vi "DeriveParameters.vi"(8 "error in (no error)":errorcluster, 9 "Parameters":T2={"number of planes"=4, "z step"=1.9999999999999998e-05, "pixel dwell time"=1.0000000000000001e-11, "z frequency"=10.0, "number of pixels"=100, "smooth points"=10, "smooth line"=10, "Sine\nSawtooth"=FALSE, "PointSorting"=0, "Sort Points"=FALSE, "X-pixels"=256.0, "Y-lines"=256.0, "pixelstoµm"=256.0, "zoom"=1.0, "Time offset"=1.0000000000000001e-11} {"zoom" min=0.5 step=0.1; "Y-lines" min=1 step=1; "X-pixels" min=1 step=1; "PointSorting" items=["No Difference", "Every Second Point", "Down / Up"]; "smooth line" min=1; "smooth points" min=1; "number of pixels" min=1; "z frequency" format="%_4g"; "number of planes" min=1}, 10 "DutyCluster":T1 {"Iteration" items=["first iteration", "second iteration"]}, 11 "XYZ Point coordinates (pixels)":dbl[][](array[numeric])) -> (0 "error out":errorcluster, 2 "DutyCluster":T1 {"Iteration" items=["first iteration", "second iteration"]})   [LabVIEW 2010]
uses:
  TypeDefs/DutyCluster.ctl
  TypeDefs/ParameterCluster.ctl
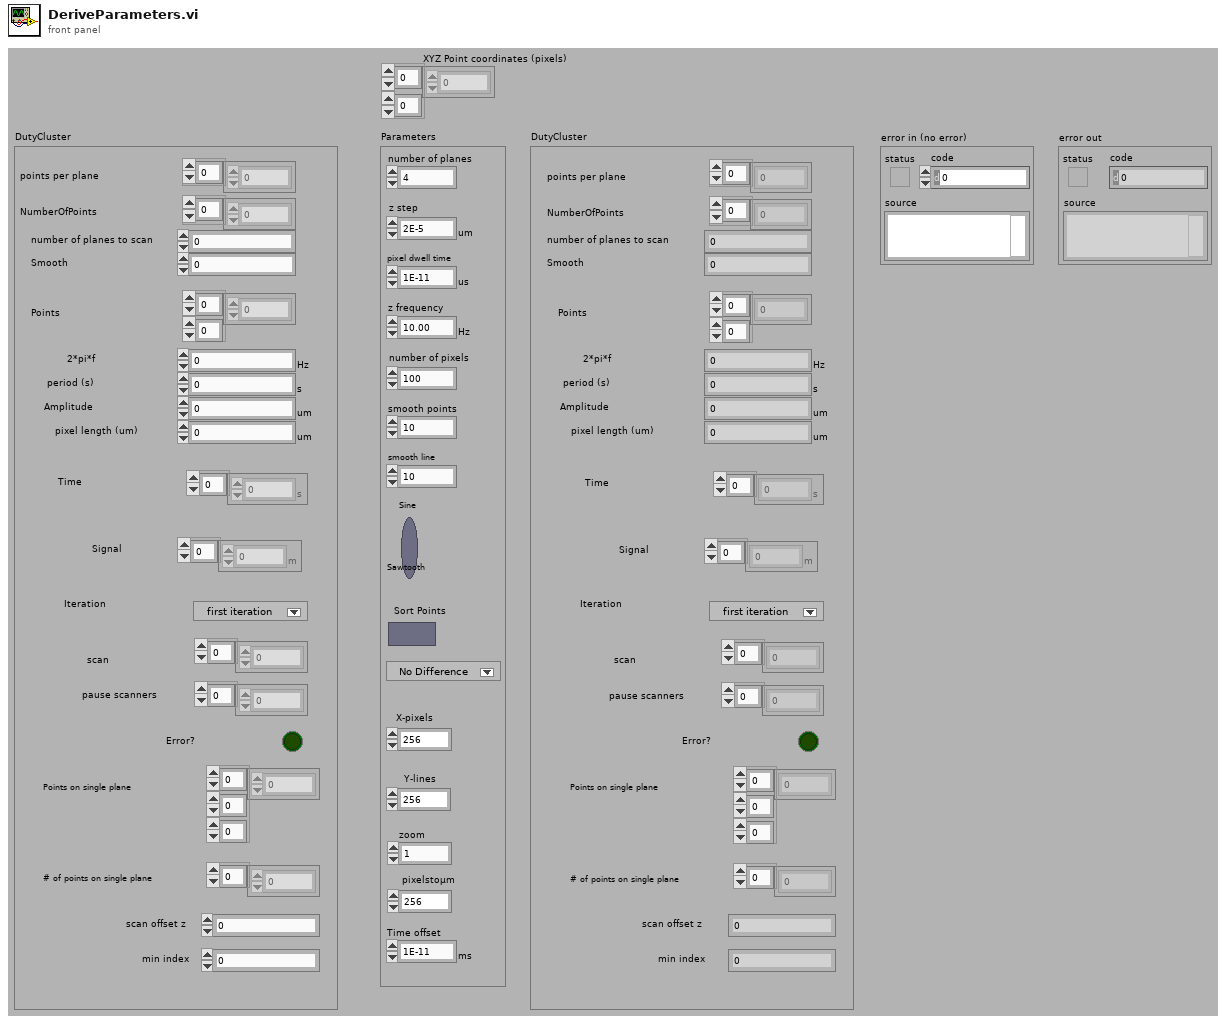
[diagram p1: front panel]
types:
  T1 = typedef "DutyCluster.ctl" = cluster{"points per plane":i32[], "NumberOfPoints":i32[], "number of planes to scan":i32, "Smooth":i32, "Points":dbl[][], "2*pi*f":dbl[unit], "period (s)":dbl[unit], "Amplitude":dbl[unit], "pixel length (um)":dbl[unit], "Time":dbl[unit][], "Signal":dbl[unit][], "Iteration":u16, "scan":i32[], "pause scanners":i32[], "Error?":bool, "Points on single plane":dbl[][][], "# of points on single plane":i32[], "scan offset z":i32, "min index":i32}
  T2 = typedef "ParameterCluster.ctl" = cluster{"number of planes":i32, "z step":dbl[unit], "pixel dwell time":dbl[unit], "z frequency":dbl[unit], "number of pixels":i32, "smooth points":i32, "smooth line":i32, "Sine\nSawtooth":bool, "PointSorting":u16, "Sort Points":bool, "X-pixels":sgl, "Y-lines":sgl, "pixelstoµm":dbl, "zoom":dbl, "Time offset":dbl[unit]}
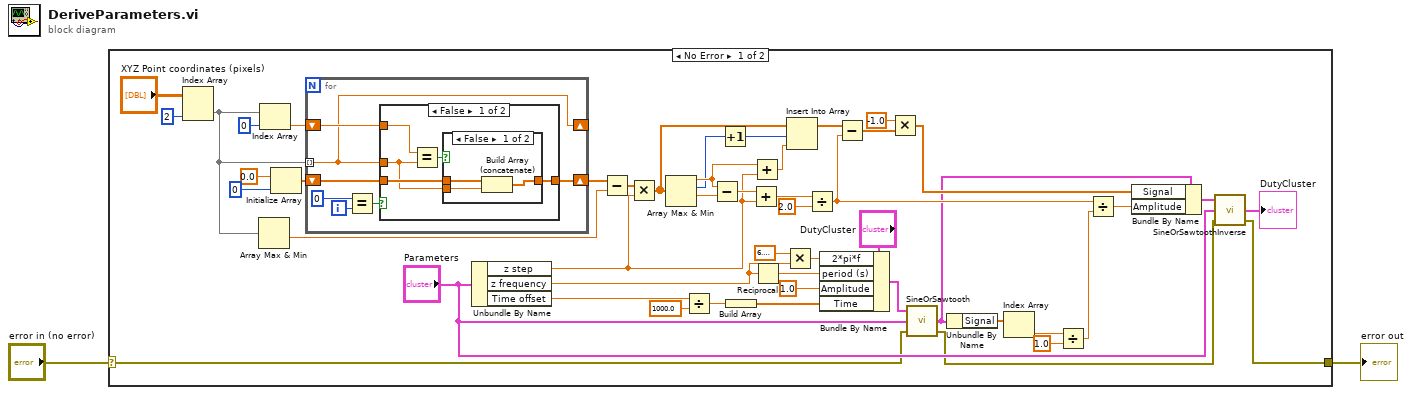
[diagram p0: block diagram]
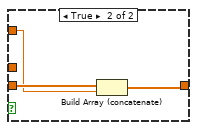
[diagram p3: hidden frame]
diagram:
  n1 = case shown="No Error" "error in (no error)" {
    selector: "error in (no error)" -> [w8 w71]
    tunnel: [w7 w71] -> w1
    frame No Error {
      n2 = Index Array(array="XYZ Point coordinates (pixels)", index (col)=2 ("disabled index (col)")) -> (element=w4:dbl[])  [unwired: 1 in]
      n3 = Array Max & Min(array=w4) -> (min value=w28:dbl)  [unwired: 3 out]
      n4 = Index Array(array=w4, index=0) -> (element=w47:dbl)
      n5 = Initialize Array(0.0 ("element"), 0 ("dimension size")) -> (w49:dbl[])
      n6 = for {
        tunnel: w4 -> [w52] mode=indexing
        shift-right: [w52] -> _
        shift-left: w47 -> [w56]
        shift-right: [w57] -> w3
        shift-left: w49 -> [w58]
        i -> [w55]
        n7 = Equal?(x=0, y=w55) -> (x = y?=w53:bool)
        n8 = case shown="False" w53 {
          tunnel: w58 -> [w62 w70]
          tunnel: [w61 w68] -> w57
          tunnel: w56 -> [w60 w69]
          tunnel: w52 -> [w59 _]
          frame False {
            n9 = Equal?(x=w60, y=w59) -> (x = y?=w63:bool)
            n10 = case shown="False" w63 {
              tunnel: w62 -> [w65 w67]
              tunnel: [w64 w67] -> w61
              tunnel: w59 -> [w66 _]
              frame False {
                n11 = Build Array (concatenate)(w65, w66) -> (w64:dbl[])
              }
              frame True {
              }
            }
          }
          frame True {
            n12 = Build Array (concatenate)(w70, w69) -> (w68:dbl[])
          }
        }
      }
      n13 = Unbundle By Name("Parameters") -> ("z step"=w27:dbl[unit], "z frequency"=w26:dbl[unit], "Time offset"=w25:dbl[unit])
      n14 = Subtract(x=w3, y=w28) -> (x-y=w31:dbl[])
      n15 = Multiply(x=w31, y=w27) -> (x*y=w39:dbl[unit][])
      n16 = Array Max & Min(array=w39) -> (max value=w38:dbl[unit], max index (indices)=w36:i32, min value=w46:dbl[unit])  [unwired: 1 out]
      n17 = Divide(x=w25, y=1000.0) -> (x/y=w30:dbl[unit])
      n18 = Subtract(x=w38, y=w46) -> (x-y=w41:dbl[unit])
      n19 = Increment(x=w36) -> (x+1=w37:i32)
      n20 = Build Array(w30) -> (w10:dbl[unit][])
      n21 = Add(x=w41, y=w27) -> (x+y=w42:dbl[unit])
      n22 = Add(x=w38, y=w27) -> (x+y=w35:dbl[unit])
      n23 = Reciprocal(x=w26) -> (1/x=w24:dbl[unit])
      n24 = Multiply(x=6.283185307179586, y=w26) -> (x*y=w23:dbl[unit])
      n25 = Insert Into Array(array=w39, index=w37, new element=w35) -> (w34:dbl[unit][])
      n26 = Divide(x=w42, y=2.0) -> (x/y=w40:dbl[unit])
      n27 = Bundle By Name(cluster="DutyCluster", "2*pi*f"=w23, "period (s)"=w24, "Amplitude"=dbl[unit] 1.0, "Time"=w10) -> (w12:T1)
      n28 = Subtract(x=w34, y=w40) -> (x-y=w32:dbl[unit][])
      n29 = Multiply(x=-1.0 ("y"), y=w32) -> (x*y=w16:dbl[unit][])
      n30 = call "SineOrSawtooth.vi"("error in (no error)"=w8, "Parameters"="Parameters", "DutyCluster"=w12) -> ("error out"=w9:errorcluster, "DutyCluster"=w5:T1)  [unwired: 1 in]
      n31 = Unbundle By Name(w5) -> ("Signal"=w17:dbl[unit][])
      n32 = Index Array(array=w17) -> (element=w19:dbl[unit])  [unwired: 1 in]
      n33 = Divide(x=w19, y=dbl[unit] 1.0) -> (x/y=w18:dbl)
      n34 = Divide(x=w40, y=w18) -> (x/y=w22:dbl[unit])
      n35 = Bundle By Name(cluster=w5, "Signal"=w16, "Amplitude"=w22) -> (w15:T1)
      n36 = call "SineOrSawtoothInverse.vi"("error in (no error)"=w9, "Parameters"="Parameters", "DutyCluster"=w15) -> ("error out"=w7:errorcluster, "DutyCluster"=→"DutyCluster":T1)  [unwired: 1 in]
    }
    frame Error {
    }
  }
  "error out" <- w1
